vi "Ke2000 Single Reading.vi"(8 "error in (no error)":errorcluster, 11 "VISA resource name":refnum<visa-resource-name>) -> (0 "error out":errorcluster, 1 "Units":string, 2 "Measurement":dbl, 3 "VISA resource name out":refnum<visa-resource-name>, 5 "uA":string)   [LabVIEW 2012]
panel:
  out "Channel":i32
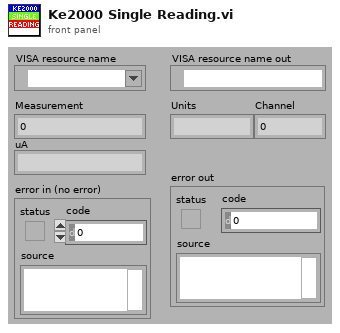
[diagram p1: front panel]
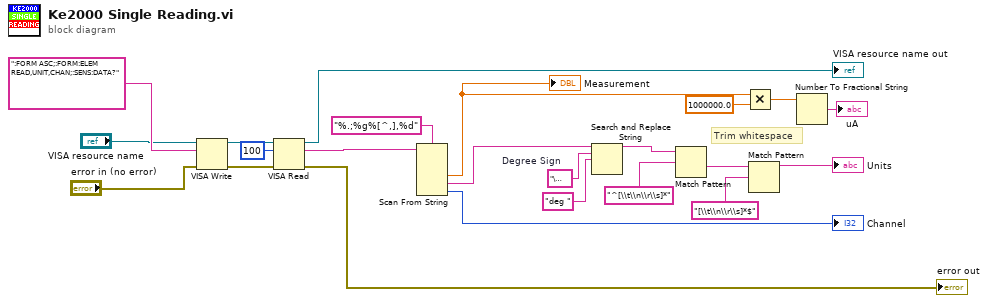
[diagram p0: block diagram]
diagram:
  w9 = "\u0013"  # Degree Sign
  # "Trim whitespace"
  n1 = VISA Write(VISA resource name="VISA resource name", write buffer=":FORM ASC;:FORM:ELEM READ,UNIT,CHAN;:SENS:DATA?", error in (no error)="error in (no error)") -> (VISA resource name out=w22:refnum<visa-resource-name>, error out=w21:errorcluster)  [unwired: 1 out]
  n2 = VISA Read(VISA resource name=w22, byte count=u32 100, error in (no error)=w21) -> (VISA resource name out=→"VISA resource name out":refnum<visa-resource-name>, read buffer=w7:string, error out=→"error out":errorcluster)  [unwired: 1 out]
  n3 = Scan From String(format string="%.;%g%[^,],%d", input string=w7) -> (output 1=w4:dbl, output 2=w10:string, output 3=→"Channel":i32)  [unwired: 5 in, 3 out]
  "Measurement" <- w4
  n4 = Search and Replace String(input string=w10, search string=w9, replace string="deg " ("replace string (\"\")")) -> (result string=w16:string)  [unwired: 5 in, 3 out]
  n5 = Match Pattern(string=w16, regular expression="^[\\t\\n\\r\\s]*") -> (after substring=w13:string)  [unwired: 1 in, 3 out]
  n6 = Multiply(x=w4, y=1000000.0) -> (x*y=w2:dbl)
  n7 = Match Pattern(string=w13, regular expression="[\\t\\n\\r\\s]*$") -> (before substring=→"Units":string)  [unwired: 1 in, 3 out]
  n8 = Number To Fractional String(number=w2) -> (F-format string=→"uA":string)  [unwired: 3 in]
